vi "Get zero pressure.vi"(8 "error in (no error)":errorcluster, 11 "Pressure Control in":refnum<class "Pressure Control.lvclass">) -> (0 "error out":errorcluster, 2 "Zero pressure level":dbl, 3 "Pressure Control out":refnum<class "Pressure Control.lvclass">)   [LabVIEW 2014, in "Pressure Control.lvclass"]
uses:
  Pressure Control.lvclass
  Pressure Control.lvclass/Pressure Control.ctl
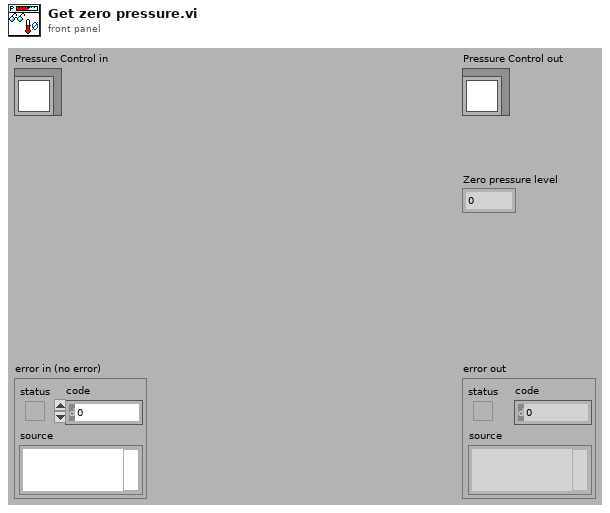
[diagram p1: front panel]
types:
  T1 = typedef "Pressure Control.lvclass/Pressure Control Status Data.ctl" = cluster{"Zero pressure level":dbl}
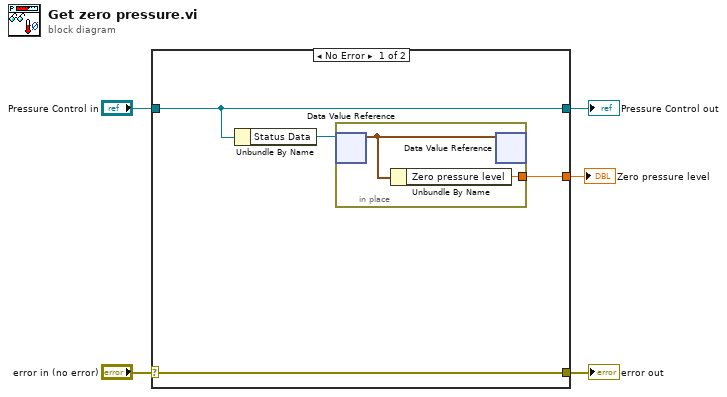
[diagram p0: block diagram]
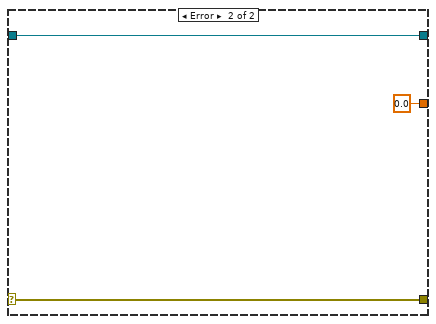
[diagram p2: hidden frame]
diagram:
  n1 = case shown="No Error" "error in (no error)" {
    selector: "error in (no error)" -> [w7 w14]
    tunnel: [w7 w14] -> w4
    tunnel: [w9 w13] -> w2
    tunnel: "Pressure Control in" -> [w9 w13]
    tunnel: [w6 0.0 ("Pressure")] -> w1
    frame No Error {
      n2 = Unbundle By Name(w9) -> ("Status Data"=w8:refnum<data-value>)
      n3 = in-place {
        in-place-border: [w10] -> w6
        n4 = in-place-dvr #1(w8) -> (w11:T1)  [unwired: 1 out]
        n5 = Unbundle By Name(w11) -> ("Zero pressure level"=w10:dbl)
        n6 = in-place-dvr #1(w11) -> ()  [unwired: 2 out]
      }
    }
    frame Error {
    }
  }
  "error out" <- w4
  "Pressure Control out" <- w2
  "Zero pressure level" <- w1
